vi "Bytes to Lowercase Hex String.vi"(1 "bytes":u8[](array[numeric]) format="%02x") -> (0 "hex string":string)   [LabVIEW 2020, in "NI_Bit Manipulation.lvlib"]
doc: "Formats a byte array as a hexadecimal string."
uses:
  <vilib>/Bit Manipulation/NI_Bit Manipulation.lvlib
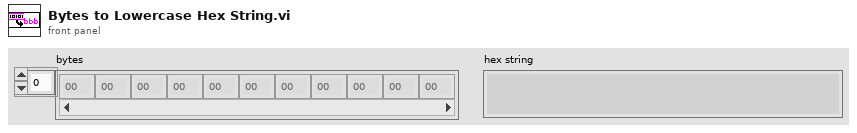
[diagram p1: front panel]
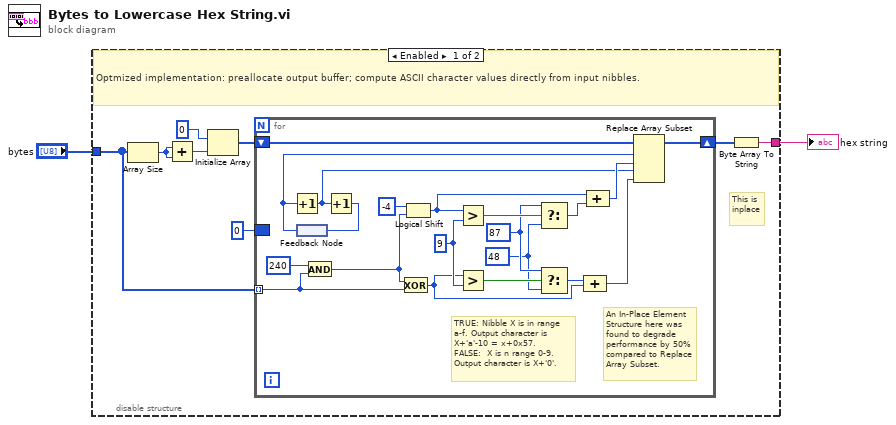
[diagram p0: block diagram]
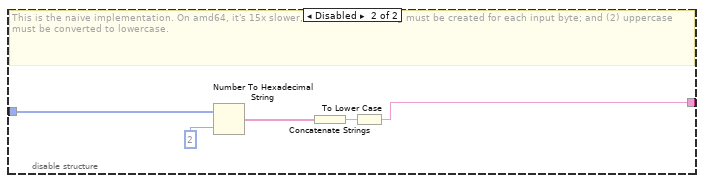
[diagram p2: hidden frame]
diagram:
  n1 = disable-structure shown="Enabled" {
    disable-tunnel: "bytes" -> [w10 w32]
    disable-tunnel: [w9 w31] -> w1
    frame Enabled {
      # "This is inplace"
      # "Optmized implementation: preallocate output buffer; compute ASCII character values directly from input nibbles."
      n2 = Array Size(array=w10) -> (size(s)=w8:i32)
      n3 = Add(x=w8, y=w8) -> (x+y=w7:i32)
      n4 = Initialize Array(u8 0, w7) -> (w5:u8[])
      n5 = for {
        shift-right: [w28] -> w4
        shift-left: w5 -> [w29]
        tunnel: w10 -> [w30] mode=indexing
        border: 0 -> [_]
        w15 = u8 48
        w16 = u8 87
        w19 = u8 9 ("x")
        # "An In-Place Element Structure here was found to degrade performance by 50% compared to Replace Array Subset."
        # "TRUE: Nibble X is in range a-f. Output character is X+'a'-10 = x+0x57.\nFALSE:  X is n range 0-9. Output character is X+'0'."
        n6 = feedback #1() -> (w27:i32)
        n7 = Increment(x=w27) -> (x+1=w12:i32)
        n8 = And(x=u8 240, y=w30) -> (x .and. y?=w14:u8)
        n9 = Increment(x=w12) -> (x+1=w11:i32)
        n10 = feedback-in #1(w11) -> ()
        n11 = Exclusive Or(1:w30, 2:w14) -> (0:w13:u8)
        n12 = Logical Shift(y=i16 -4, x=w14) -> (x << y=w23:u8)
        n13 = Greater?(x=w23, y=w19) -> (0:w18:bool)
        n14 = Greater?(x=w13, y=w19) -> (0:w17:bool)
        n15 = Select(t=w16, s=w18, f=w15) -> (s? t:f=w24:u8)
        n16 = Select(t=w16, s=w17, f=w15) -> (s? t:f=w21:u8)
        n17 = Compound Arithmetic op=ADD(w21, w13) -> (w20:u8)
        n18 = Compound Arithmetic op=ADD(w23, w24) -> (w22:u8)
        n19 = Replace Array Subset(array=w29, new element #1=w22, index #1=w27, new element #2=w20, index #2=w12) -> (w28:u8[])
      }
      n20 = Byte Array To String(unsigned byte array=w4) -> (string=w9:string)
    }
    frame Disabled {
      # "This is the naive implementation. On amd64, it's 15x slower, because (1) a string must be created for each input byte; and (2) uppercase must be converted to lowercase."
      n21 = Number To Hexadecimal String(1:i16 2 ("width (-)"), 2:w32) -> (0:w34:string[])
      n22 = Concatenate Strings(w34) -> (w35:string)
      n23 = To Lower Case(string=w35) -> (all lower case string=w31:string)
    }
  }
  "hex string" <- w1
